vi "DFD Scale Filter.vi"(7 "scale type":T1=enum."Time Domain 1-Norm", 8 "error in (no error)":errorcluster, 11 "filter in":T2={"mSRate_Fs"=1.0, "mSRate_Version"="2.0", "mSRate_Comments"="", "mSRate_OrgCoef"={"type"=enum."Undefined", "gain"=1.0, "coef a (k)"=[], "coef b (v)"=[]}, "mSRate_CurCoef"={"type"=enum."Undefined", "gain"=1.0, "coef a (k)"=[], "coef b (v)"=[]}, "mSRate_Quantized?"=FALSE, "mSRate_QCoef"={"type"=enum."Undefined", "gain"=1.0, "coef a (k)"=[], "coef b (v)"=[]}, "mSRate_QSettings"=[], "mSRate_Order"=0, "mSRate_Scaling"={"mSRate_ScaleByPowerOf2?"=FALSE, "mSRate_ScaleType"=enum."No Norm"}} {"mSRate_QSettings"."source" items=["Coef a/k"=0, "Coef b/v"=7, "Input"=1, "Output"=2, "Multiplicand"=3, "Product"=4, "Sum"=5, "Delay"=6, "Gain"=8]}) -> (0 "error out":errorcluster, 3 "filter out":T2={"mSRate_Fs"=1.0, "mSRate_Version"="2.0", "mSRate_Comments"="", "mSRate_OrgCoef"={"type"=enum."Undefined", "gain"=1.0, "coef a (k)"=[], "coef b (v)"=[]}, "mSRate_CurCoef"={"type"=enum."Undefined", "gain"=1.0, "coef a (k)"=[], "coef b (v)"=[]}, "mSRate_Quantized?"=FALSE, "mSRate_QCoef"={"type"=enum."Undefined", "gain"=1.0, "coef a (k)"=[], "coef b (v)"=[]}, "mSRate_QSettings"=[], "mSRate_Order"=0, "mSRate_Scaling"={"mSRate_ScaleByPowerOf2?"=FALSE, "mSRate_ScaleType"=enum."No Norm"}} {"mSRate_QSettings"."source" items=["Coef a/k"=0, "Coef b/v"=7, "Input"=1, "Output"=2, "Multiplicand"=3, "Product"=4, "Sum"=5, "Delay"=6, "Gain"=8]})   [LabVIEW 2017, in "NI_DigFilterLicensed.lvlib"]
doc: "Scales the coefficients of a filter without changing the characteristics of the filter."
uses:
  <vilib>/addons/Digital Filter Design/NI_DigFilterLicensed.lvlib
  <vilib>/addons/Digital Filter Design/_Objects.llb/DFD Filter Obj.ctl
  <vilib>/addons/Digital Filter Design/_Objects.llb/DFD Filter Coef.ctl
  <vilib>/addons/Digital Filter Design/_Objects.llb/DFD Filter Structure Type Selector.ctl
  <vilib>/addons/Digital Filter Design/_Objects.llb/dfd_Internal Quantization Settings.ctl
  <vilib>/addons/Digital Filter Design/_Objects.llb/dfd_Internal Quantization Srcs.ctl
  <vilib>/addons/Digital Filter Design/_Objects.llb/DFD Coef Norm Type.ctl
  <vilib>/addons/Digital Filter Design/NI_DigFilter_FXP.lvlib
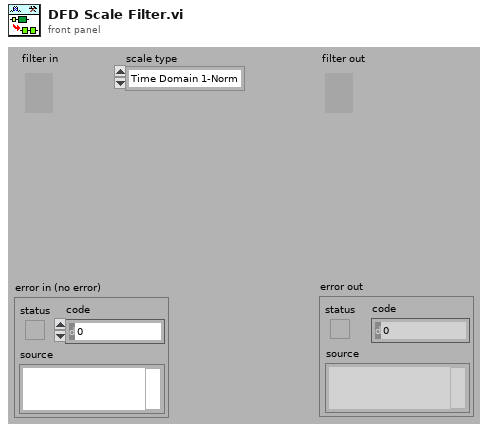
[diagram p1: front panel]
types:
  T1 = typedef "NI_DigFilterLicensed.lvlib/DFD Coef Norm Type.ctl" = enum16{"No Norm", "Time Domain 1-Norm", "Time Domain 2-Norm", "Time Domain Inf-Norm"}
  T2 = typedef "NI_DigFilterLicensed.lvlib/DFD Filter Obj.ctl" = cluster{"mSRate_Fs":dbl, "mSRate_Version":string, "mSRate_Comments":string, "mSRate_OrgCoef":T3, "mSRate_CurCoef":T3, "mSRate_Quantized?":bool, "mSRate_QCoef":T3, "mSRate_QSettings":T5[], "mSRate_Order":i32, "mSRate_Scaling":cluster{"mSRate_ScaleByPowerOf2?":bool, "mSRate_ScaleType":T1}}
  T3 = typedef "NI_DigFilterLicensed.lvlib/DFD Filter Coef.ctl" = cluster{"type":T4, "gain":dbl, "coef a (k)":dbl[], "coef b (v)":dbl[]}
  T4 = typedef "NI_DigFilterLicensed.lvlib/DFD Filter Structure Type Selector.ctl" = enum16{"Undefined", "FIR Direct Form", "FIR Direct Form Transposed", "FIR Symmetric", "FIR Antisymmetric", "IIR Direct Form I", "IIR Direct Form I Transposed", "IIR Direct Form II", "IIR Direct Form II Transposed", "IIR Cascaded Second Order Sections Form I", "IIR Cascaded Second Order Sections Form I Transposed", "IIR Cascaded Second Order Sections Form II", "IIR Cascaded Second Order Sections Form II Transposed", "Lattice Allpass (basic sections)", "Lattice Allpass (one multiplier sections)", "Lattice Allpass (normalized sections)", "Lattice AR (basic sections)", "Lattice AR (one multiplier sections)", "Lattice AR (normalized sections)", "Lattice MA (minimum phase)", "Lattice MA (maximum phase)", "Lattice ARMA (basic sections)", "Lattice ARMA (one multiplier sections)", "Lattice ARMA (normalized sections)"}
  T5 = typedef "NI_DigFilterLicensed.lvlib/dfd_Internal Quantization Settings.ctl" = cluster{"source":T6, "wl":i16, "iwl":i16, "overflow mode":enum16{"Saturation", "Wrap"}, "rounding mode":enum16{"Nearest", "Truncation"}, "signed?":bool}
  T6 = typedef "NI_DigFilterLicensed.lvlib/dfd_Internal Quantization Srcs.ctl" = u16
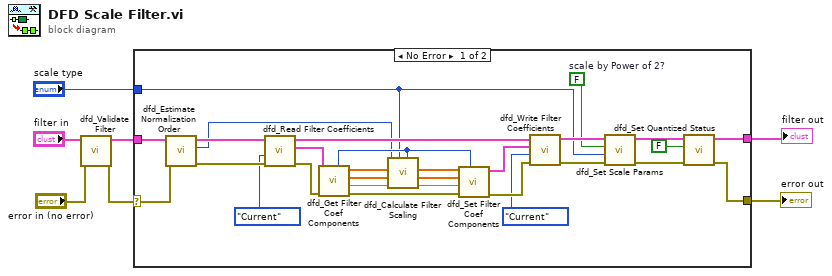
[diagram p0: block diagram]
diagram:
  n1 = call <vilib>:"dfd_Validate Filter.vi"("error in (no error)"="error in (no error)", "filter in"="filter in") -> ("error out"=w1:errorcluster, "filter out"=w4:T2)  [unwired: 1 in, 7 out]
  n2 = case shown="No Error" w1 {
    selector: w1 -> [w14 w36]
    tunnel: w4 -> [w23 w37]
    tunnel: [w17 w37] -> w7
    tunnel: [w16 w36] -> w6
    tunnel: "scale type" -> [w9 _]
    frame No Error {
      w8 = FALSE  # scale by Power of 2?
      n3 = call <vilib>:"dfd_Estimate Normalization Order.vi"("error in (no error)"=w14, "filter in"=w23) -> ("error out"=w21:errorcluster, "iteration"=w19:i32, "filter out"=w22:T2)  [unwired: 7 out]
      n4 = call <vilib>:"dfd_Read Filter Coefficients.vi"("error in (no error)"=w21, "coef source"=enum16{"Original", "Current", "Quantized"}."Current", "filter in"=w22) -> ("error out"=w18:errorcluster, "filter coef"=w35:T3, "filter out"=w27:T2)  [unwired: 6 out]
      n5 = call <vilib>:"dfd_Get Filter Coef Components.vi"("error in (no error)"=w18, "filter coef"=w35) -> ("error out"=w25:errorcluster, "gain"=w32:dbl, "coef a (k)"=w33:dbl[], "coef b (v)"=w34:dbl[], "type"=w28:T4)  [unwired: 5 out]
      n6 = call <vilib>:"dfd_Calculate Filter Scaling.vi"("structure type"=w28, "scale type"=w9, "gain"=w32, "coef a/k"=w33, "coef b/v"=w34, "iterations"=w19) -> ("scaled gain"=w29:dbl, "scaled coefficients a/k"=w30:dbl[], "scaled coefficients b/v"=w31:dbl[])  [unwired: 3 out]
      n7 = call <vilib>:"dfd_Set Filter Coef Components.vi"("type"=w28, "error in (no error)"=w25, "gain"=w29, "coef a (k)"=w30, "coef b (v)"=w31) -> ("error out"=w24:errorcluster, "filter coef"=w26:T3)  [unwired: 5 out]
      n8 = call <vilib>:"dfd_Write Filter Coefficients.vi"("error in (no error)"=w24, "coef source"=enum16{"Original", "Current", "Quantized"}."Current", "filter coef"=w26, "filter in"=w27) -> ("error out"=w10:errorcluster, "filter out"=w12:T2)  [unwired: 6 out]
      n9 = call <vilib>:"dfd_Set Scale Params.vi"("scale type"=w9, "scale by Power of 2?"=w8, "filter in"=w12) -> ("filter out"=w11:T2)  [unwired: 8 out]
      n10 = call <vilib>:"dfd_Set Quantized Status.vi"("error in (no error)"=w10, "quantized?"=FALSE, "filter in"=w11) -> ("error out"=w16:errorcluster, "filter out"=w17:T2)  [unwired: 7 out]
    }
    frame Error {
    }
  }
  "filter out" <- w7
  "error out" <- w6
